vi "split string.vi"(10 "tokens":T4[](array[typedef]), 11 "String":string) -> (3 "layers":T1[](array[typedef]))   [LabVIEW 2013]
uses:
  json token.ctl
  json node type.ctl
  layer.ctl
  processed node.ctl
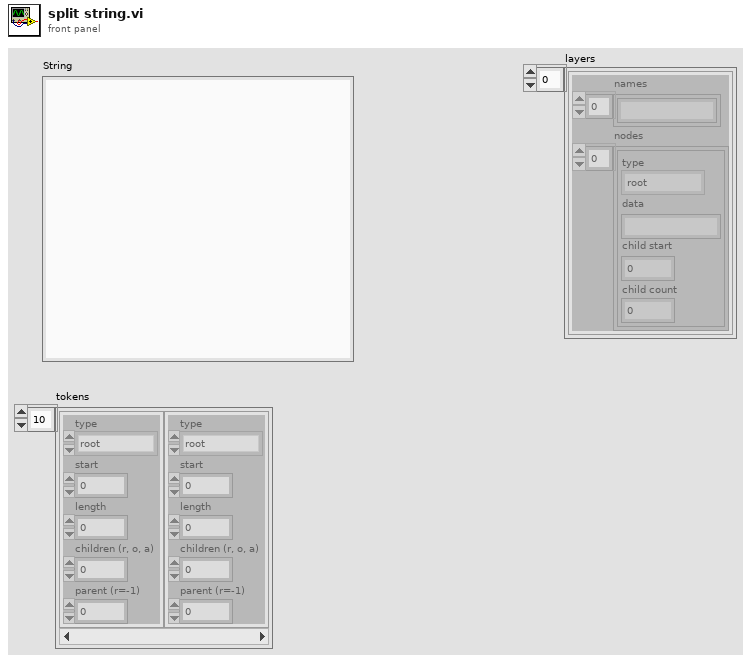
[diagram p1: front panel]
types:
  T1 = typedef "layer.ctl" = cluster{"names":string[], "nodes":T2[]}
  T2 = typedef "processed node.ctl" = cluster{"type":T3, "data":string, "child start":i32, "child count":i32}
  T3 = typedef "json node type.ctl" = enum16{"root", "object", "array", "number", "string value", "string key", "true", "false", "null"}
  T4 = typedef "json token.ctl" = cluster{"type":T3, "start":i32, "length":i32, "children (r, o, a)":u16, "parent (r=-1)":i32}
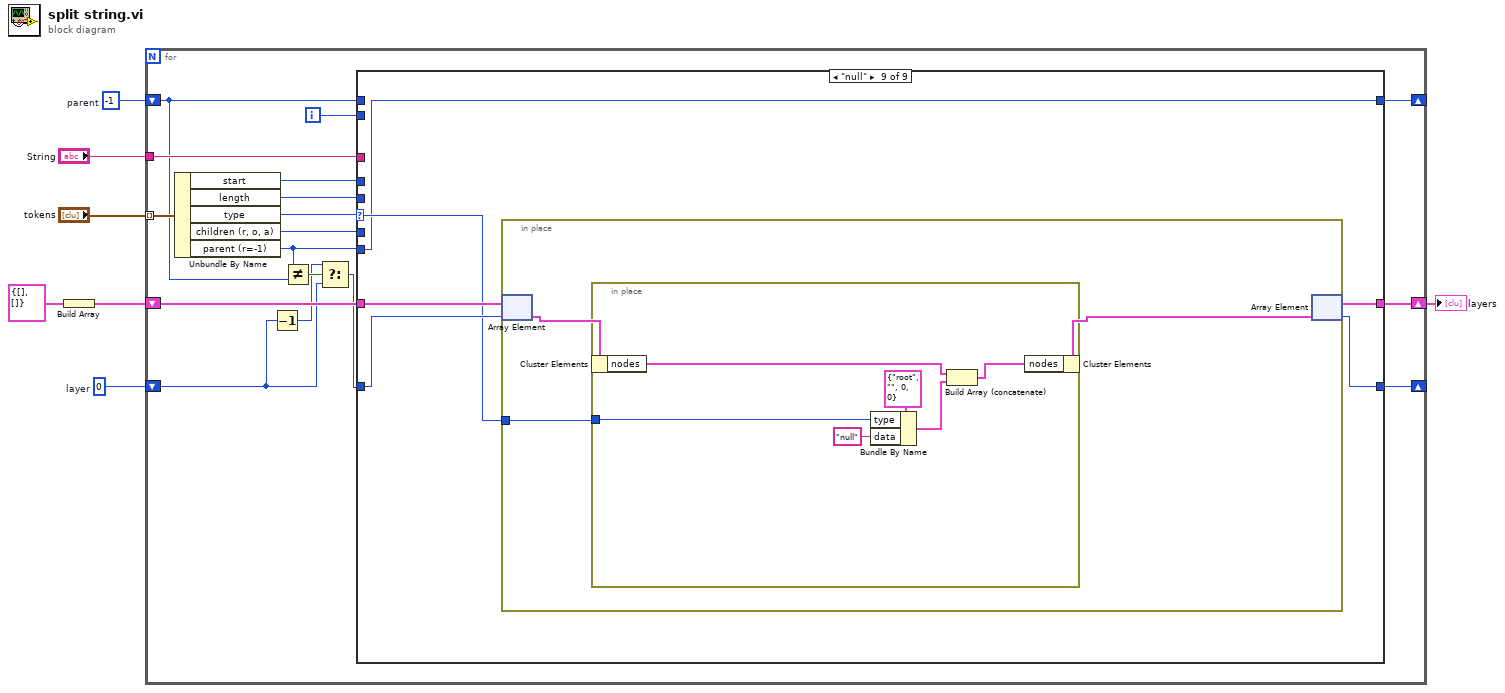
[diagram p0: block diagram]
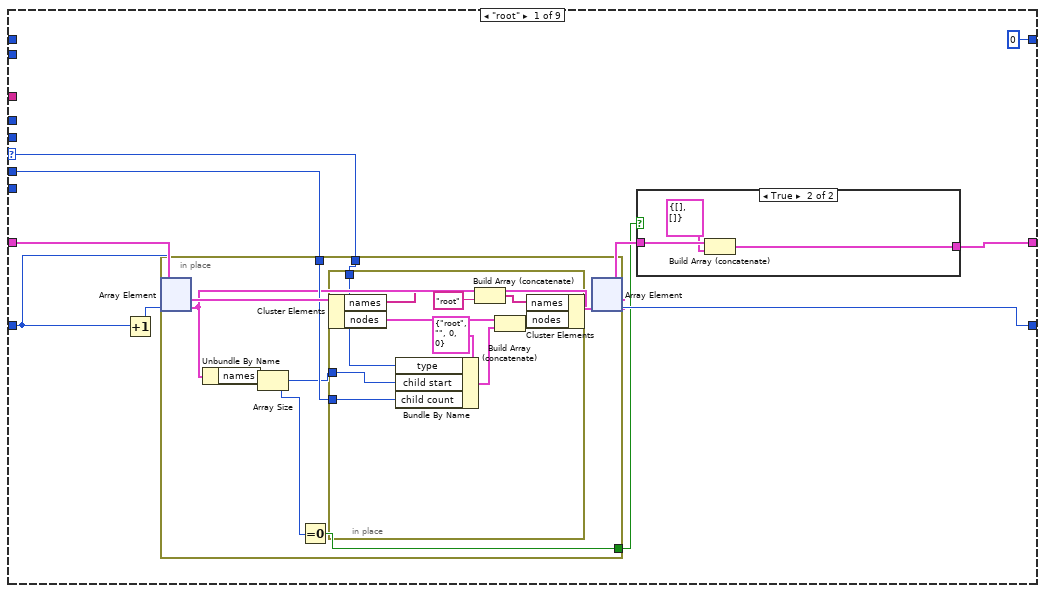
[diagram p2: hidden frame]
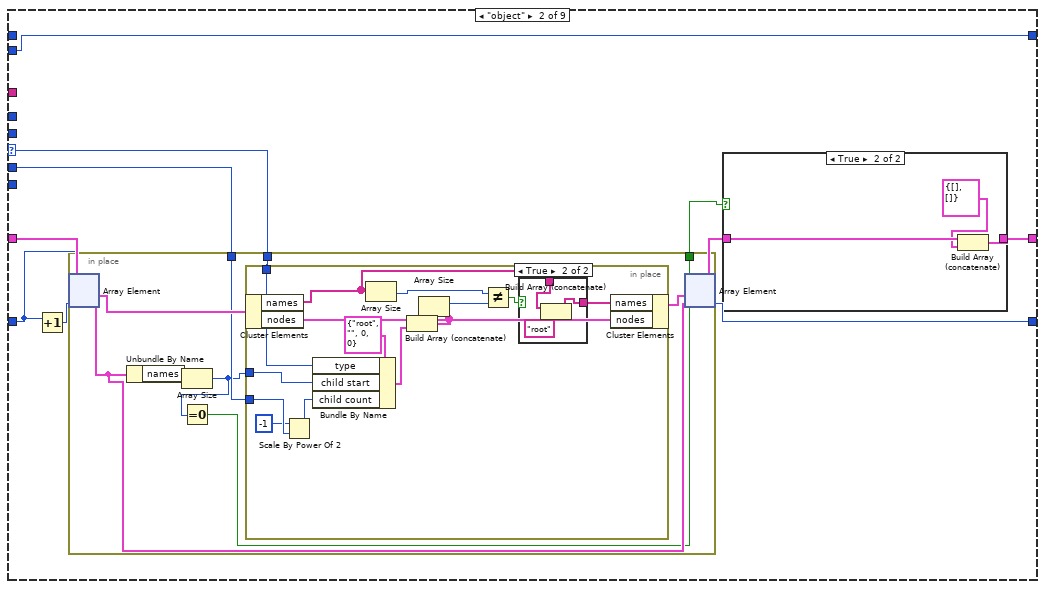
[diagram p4: hidden frame]
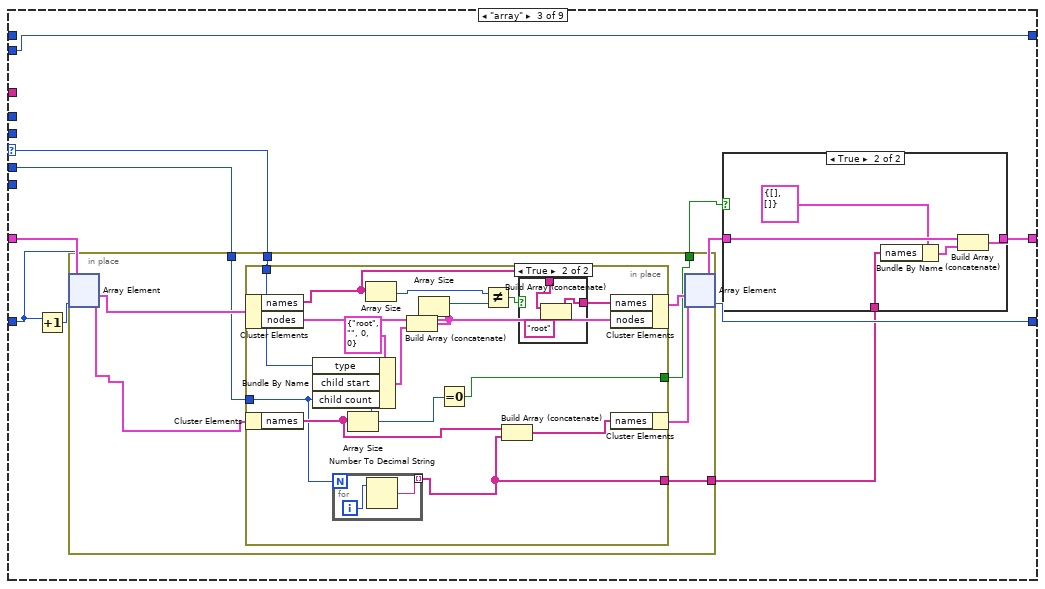
[diagram p7: hidden frame]
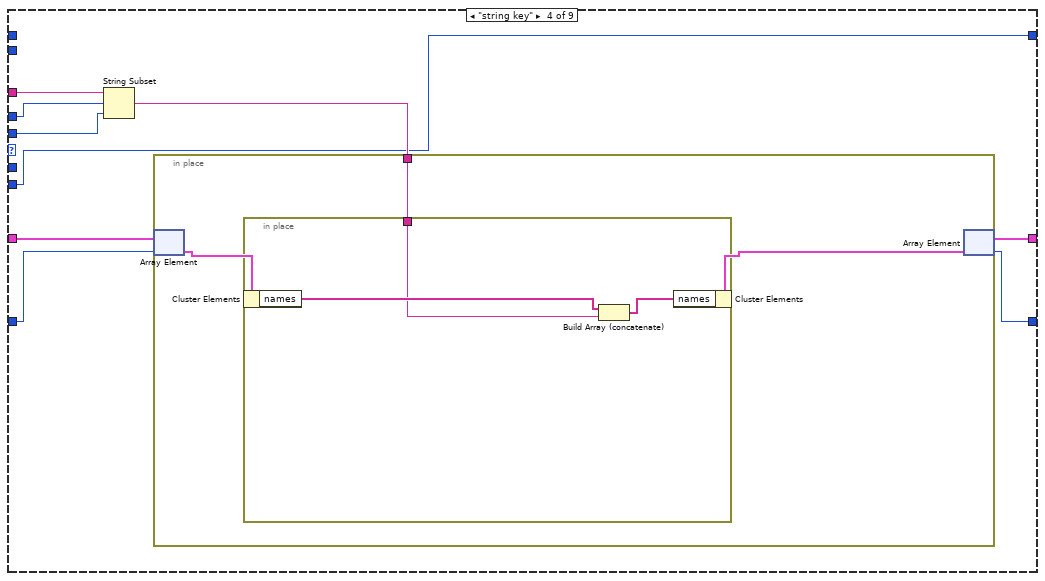
[diagram p10: hidden frame]
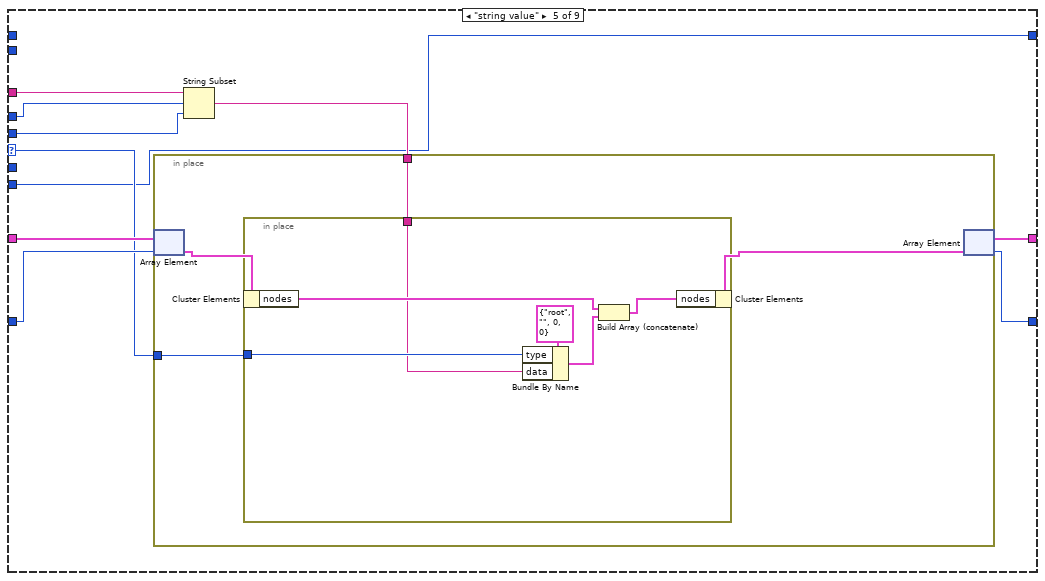
[diagram p11: hidden frame]
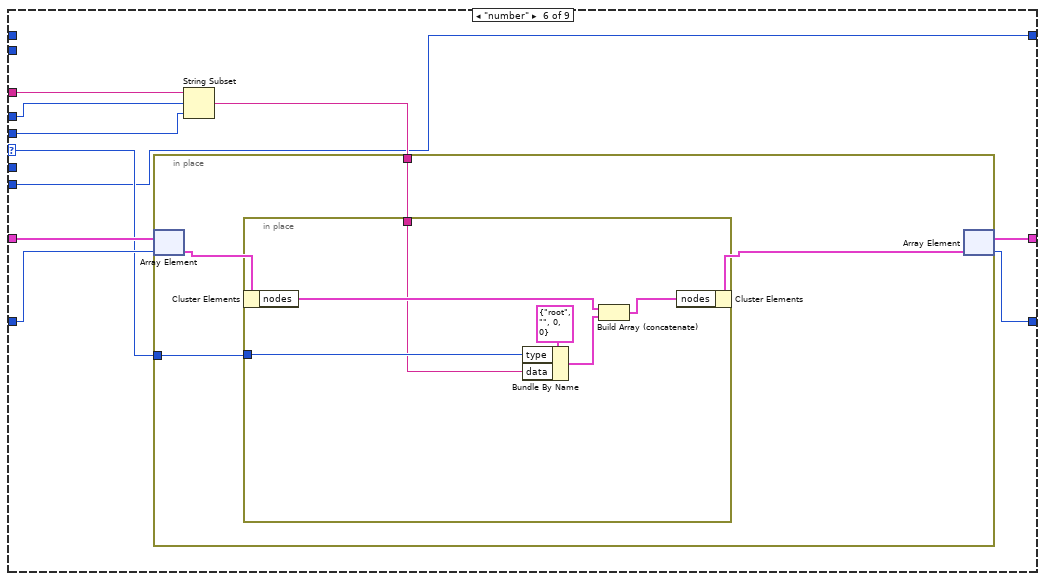
[diagram p12: hidden frame]
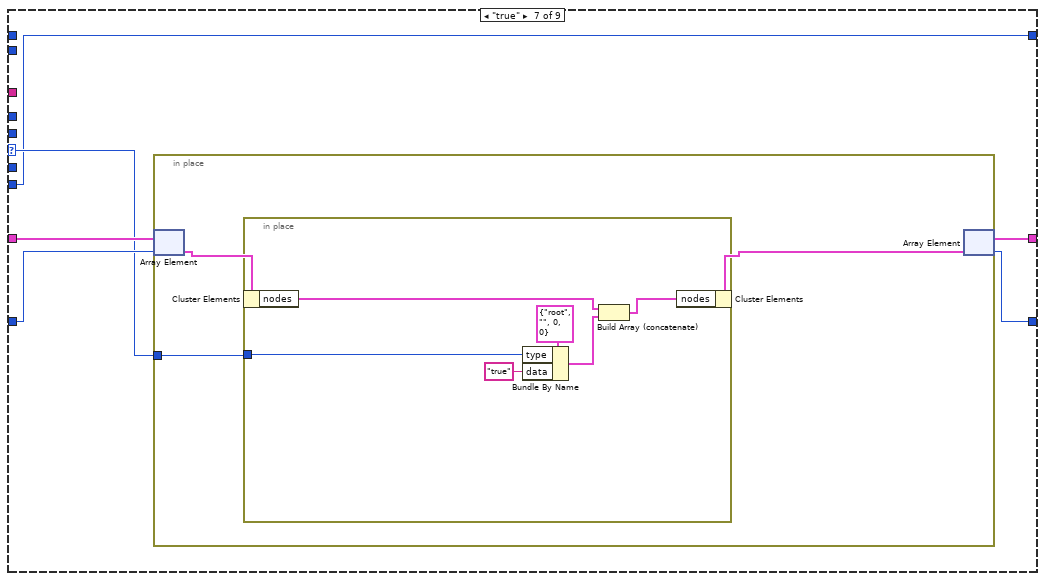
[diagram p13: hidden frame]
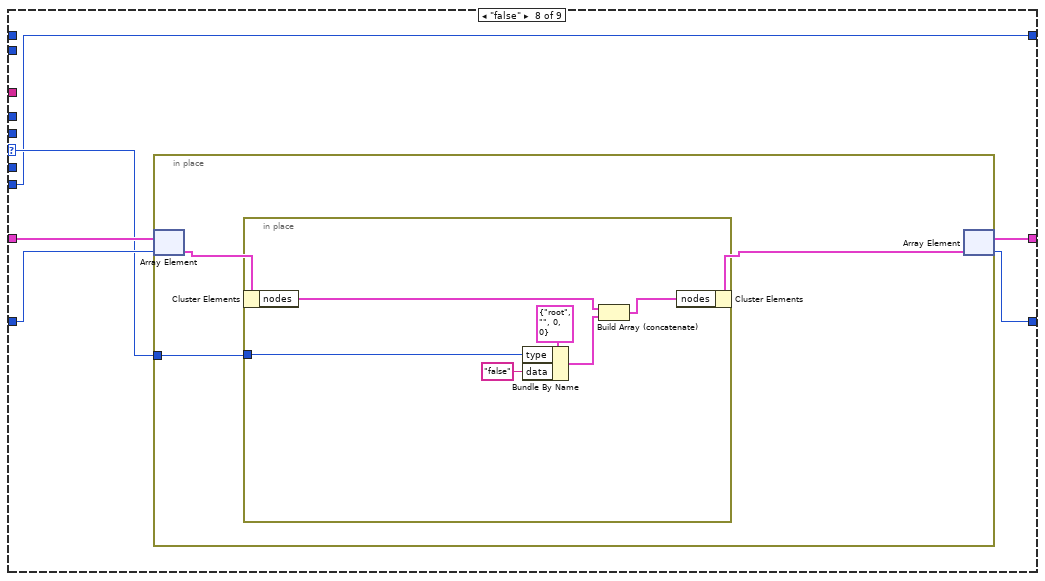
[diagram p14: hidden frame]
diagram:
  w3 = -1  # parent
  w4 = 0  # layer
  n1 = Build Array(T1 {"names"=[], "nodes"=[]} ("layer")) -> (w1:T1[])
  n2 = for {
    tunnel: "tokens" -> [w24] mode=indexing
    tunnel: "String" -> [w22]
    shift-right: [w17] -> w5
    shift-left: w1 -> [w18]
    shift-right: [w16] -> _
    shift-left: w4 -> [w10]
    shift-right: [w15] -> _
    shift-left: w3 -> [w13]
    i -> [w8]
    n3 = Unbundle By Name(w24) -> ("start"=w21:i32, "length"=w19:i32, "type"=w23:T3, "children (r, o, a)"=w20:u16, "parent (r=-1)"=w14:i32)
    n4 = Decrement(x=w10) -> (x-1=w11:i32)
    n5 = Not Equal?(x=w14, y=w13) -> (x != y?=w12:bool)
    n6 = Select(t=w11, s=w12, f=w10) -> (s? t:f=w9:i32)
    n7 = case shown="\"null\"" w23 {
      selector: w23 -> [w29 w61 w102 _ w164 w184 w200 w215 w230]
      tunnel: w22 -> [_ _ _ w148 w163 w183 _ _ _]
      tunnel: w21 -> [_ _ _ w147 w162 w182 _ _ _]
      tunnel: w20 -> [w28 w60 w101 _ _ _ _ _ _]
      tunnel: w19 -> [_ _ _ w146 w161 w181 _ _ _]
      tunnel: w14 -> [_ _ _ w144 w159 w179 w199 w214 w229]
      tunnel: w18 -> [w34 w66 w107 w151 w167 w187 w203 w218 w233]
      tunnel: w9 -> [w32 w64 w105 w152 w168 w188 w204 w219 w234]
      tunnel: [w26 w58 w99 w150 w166 w186 w202 w217 w232] -> w17
      tunnel: [w30 w62 w103 w149 w165 w185 w201 w216 w231] -> w16
      tunnel: [0 ("parent") w59 w100 w144 w159 w179 w199 w214 w229] -> w15
      tunnel: w13 -> [_ _ _ _ _ _ _ _ _]
      tunnel: w8 -> [_ w59 w100 _ _ _ _ _ _]
      frame "root" {
        n8 = Increment(x=w32) -> (x+1=w31:i32)
        n9 = in-place {
          in-place-border: w29 -> [w44]
          in-place-border: w28 -> [w43]
          in-place-border: [w39] -> w25
          n10 = in-place-array #1(w34, w32, w31) -> (w46:T1, w41:T1)
          n11 = Unbundle By Name(w41) -> ("names"=w42:string[])
          n12 = Array Size(array=w42) -> (size(s)=w40:i32)
          n13 = Equal To 0?(x=w40) -> (x = 0?=w39:bool)
          n14 = in-place {
            in-place-border: w44 -> [w50]
            in-place-border: w43 -> [w48]
            in-place-border: w40 -> [w47]
            n15 = in-place-cluster #2(w46) -> ("names"=w56:string[], "nodes"=w53:T2[])
            n16 = Bundle By Name(cluster=T2 {"type"=enum."root", "data"="", "child start"=0, "child count"=0} ("node"), "type"=w50, "child start"=w47, "child count"=w48) -> (w49:T2)
            n17 = Build Array (concatenate)(w56, "root") -> (w54:string[])
            n18 = Build Array (concatenate)(w53, w49) -> (w52:T2[])
            n19 = in-place-cluster #2("names"=w54, "nodes"=w52) -> (w45:T1)
          }
          n20 = in-place-array #1(w45, w41) -> (w33:T1[], w30:i32)  [unwired: 1 out]
        }
        n21 = case shown="True" w25 {
          tunnel: w33 -> [w35 w38]
          tunnel: [w35 w37] -> w26
          frame False {
          }
          frame True {
            n22 = Build Array (concatenate)(w38, T1 {"names"=[], "nodes"=[]} ("layer")) -> (w37:T1[])
          }
        }
      }
      frame "object" {
        n23 = Increment(x=w64) -> (x+1=w63:i32)
        n24 = in-place {
          in-place-border: w61 -> [w76]
          in-place-border: w60 -> [w75]
          in-place-border: [w71] -> w57
          n25 = in-place-array #3(w66, w64, w63) -> (w78:T1, w73:T1)
          n26 = Unbundle By Name(w73) -> ("names"=w74:string[])
          n27 = Array Size(array=w74) -> (size(s)=w72:i32)
          n28 = Equal To 0?(x=w72) -> (x = 0?=w71:bool)
          n29 = in-place {
            in-place-border: w76 -> [w90]
            in-place-border: w75 -> [w81]
            in-place-border: w72 -> [w88]
            n30 = in-place-cluster #4(w78) -> ("names"=w83:string[], "nodes"=w92:T2[])
            n31 = Scale By Power Of 2(n=i16 -1, x=w81) -> (x*2^n=w80:u16)
            n32 = Bundle By Name(cluster=T2 {"type"=enum."root", "data"="", "child start"=0, "child count"=0} ("node"), "type"=w90, "child start"=w88, "child count"=w80) -> (w89:T2)
            n33 = Array Size(array=w83) -> (size(s)=w85:i32)
            n34 = Build Array (concatenate)(w92, w89) -> (w87:T2[])
            n35 = Array Size(array=w87) -> (size(s)=w86:i32)
            n36 = Not Equal?(x=w85, y=w86) -> (x != y?=w84:bool)
            n37 = case shown="True" w84 {
              tunnel: w83 -> [w93 w96]
              tunnel: [w93 w95] -> w82
              frame False {
              }
              frame True {
                n38 = Build Array (concatenate)(w96, "root") -> (w95:string[])
              }
            }
            n39 = in-place-cluster #4("names"=w82, "nodes"=w87) -> (w77:T1)
          }
          n40 = in-place-array #3(w77, w73) -> (w65:T1[], w62:i32)  [unwired: 1 out]
        }
        n41 = case shown="True" w57 {
          tunnel: w65 -> [w67 w70]
          tunnel: [w67 w69] -> w58
          frame False {
          }
          frame True {
            n42 = Build Array (concatenate)(w70, T1 {"names"=[], "nodes"=[]} ("layer")) -> (w69:T1[])
          }
        }
      }
      frame "array" {
        n43 = Increment(x=w105) -> (x+1=w104:i32)
        n44 = in-place {
          in-place-border: w102 -> [w119]
          in-place-border: w101 -> [w118]
          in-place-border: [w115] -> w98
          in-place-border: [w114] -> w97
          n45 = in-place-array #5(w107, w105, w104) -> (w121:T1, w117:T1)
          n46 = in-place {
            in-place-border: w119 -> [w135]
            in-place-border: w118 -> [w123]
            in-place-border: [w127] -> w115
            in-place-border: [w122] -> w114
            n47 = in-place-cluster #6(w121) -> ("names"=w129:string[], "nodes"=w137:T2[])
            n48 = in-place-cluster #7(w117) -> ("names"=w125:string[])
            n49 = for {
              N: w123 -> [_]
              tunnel: [w138] -> w122 mode=indexing
              i -> [w139]
              n50 = Number To Decimal String(number=w139) -> (decimal integer string=w138:string)  [unwired: 1 in]
            }
            n51 = Array Size(array=w125) -> (size(s)=w126:i32)
            n52 = Bundle By Name(cluster=T2 {"type"=enum."root", "data"="", "child start"=0, "child count"=0} ("node"), "type"=w135, "child start"=w126, "child count"=w123) -> (w134:T2)
            n53 = Array Size(array=w129) -> (size(s)=w131:i32)
            n54 = Build Array (concatenate)(w137, w134) -> (w133:T2[])
            n55 = Array Size(array=w133) -> (size(s)=w132:i32)
            n56 = Equal To 0?(x=w126) -> (x = 0?=w127:bool)
            n57 = Not Equal?(x=w131, y=w132) -> (x != y?=w130:bool)
            n58 = Build Array (concatenate)(w125, w122) -> (w124:string[])
            n59 = case shown="True" w130 {
              tunnel: w129 -> [w140 w143]
              tunnel: [w140 w142] -> w128
              frame False {
              }
              frame True {
                n60 = Build Array (concatenate)(w143, "root") -> (w142:string[])
              }
            }
            n61 = in-place-cluster #6("names"=w128, "nodes"=w133) -> (w120:T1)
            n62 = in-place-cluster #7("names"=w124) -> (w116:T1)
          }
          n63 = in-place-array #5(w120, w116) -> (w106:T1[], w103:i32)  [unwired: 1 out]
        }
        n64 = case shown="True" w98 {
          tunnel: w106 -> [w108 w113]
          tunnel: [w108 w112] -> w99
          tunnel: w97 -> [_ w109]
          frame False {
          }
          frame True {
            n65 = Bundle By Name(cluster=T1 {"names"=[], "nodes"=[]} ("layer"), "names"=w109) -> (w110:T1)
            n66 = Build Array (concatenate)(w113, w110) -> (w112:T1[])
          }
        }
      }
      frame "string key" {
        n67 = String Subset(string=w148, offset (0)=w147, length (rest)=w146) -> (substring=w145:string)
        n68 = in-place {
          in-place-border: w145 -> [w153]
          n69 = in-place-array #8(w151, w152) -> (w155:T1)
          n70 = in-place {
            in-place-border: w153 -> [w156]
            n71 = in-place-cluster #9(w155) -> ("names"=w158:string[])
            n72 = Build Array (concatenate)(w158, w156) -> (w157:string[])
            n73 = in-place-cluster #9("names"=w157) -> (w154:T1)
          }
          n74 = in-place-array #8(w154) -> (w150:T1[], w149:i32)
        }
      }
      frame "string value" {
        n75 = String Subset(string=w163, offset (0)=w162, length (rest)=w161) -> (substring=w160:string)
        n76 = in-place {
          in-place-border: w164 -> [w170]
          in-place-border: w160 -> [w169]
          n77 = in-place-array #10(w167, w168) -> (w172:T1)
          n78 = in-place {
            in-place-border: w170 -> [w174]
            in-place-border: w169 -> [w173]
            n79 = in-place-cluster #11(w172) -> ("nodes"=w176:T2[])
            n80 = Bundle By Name(cluster=T2 {"type"=enum."root", "data"="", "child start"=0, "child count"=0} ("node"), "type"=w174, "data"=w173) -> (w178:T2)
            n81 = Build Array (concatenate)(w176, w178) -> (w175:T2[])
            n82 = in-place-cluster #11("nodes"=w175) -> (w171:T1)
          }
          n83 = in-place-array #10(w171) -> (w166:T1[], w165:i32)
        }
      }
      frame "number" {
        n84 = String Subset(string=w183, offset (0)=w182, length (rest)=w181) -> (substring=w180:string)
        n85 = in-place {
          in-place-border: w184 -> [w190]
          in-place-border: w180 -> [w189]
          n86 = in-place-array #12(w187, w188) -> (w192:T1)
          n87 = in-place {
            in-place-border: w190 -> [w194]
            in-place-border: w189 -> [w193]
            n88 = in-place-cluster #13(w192) -> ("nodes"=w196:T2[])
            n89 = Bundle By Name(cluster=T2 {"type"=enum."root", "data"="", "child start"=0, "child count"=0} ("node"), "type"=w194, "data"=w193) -> (w198:T2)
            n90 = Build Array (concatenate)(w196, w198) -> (w195:T2[])
            n91 = in-place-cluster #13("nodes"=w195) -> (w191:T1)
          }
          n92 = in-place-array #12(w191) -> (w186:T1[], w185:i32)
        }
      }
      frame "true" {
        n93 = in-place {
          in-place-border: w200 -> [w205]
          n94 = in-place-array #14(w203, w204) -> (w207:T1)
          n95 = in-place {
            in-place-border: w205 -> [w209]
            n96 = in-place-cluster #15(w207) -> ("nodes"=w211:T2[])
            n97 = Bundle By Name(cluster=T2 {"type"=enum."root", "data"="", "child start"=0, "child count"=0} ("node"), "type"=w209, "data"="true") -> (w213:T2)
            n98 = Build Array (concatenate)(w211, w213) -> (w210:T2[])
            n99 = in-place-cluster #15("nodes"=w210) -> (w206:T1)
          }
          n100 = in-place-array #14(w206) -> (w202:T1[], w201:i32)
        }
      }
      frame "false" {
        n101 = in-place {
          in-place-border: w215 -> [w220]
          n102 = in-place-array #16(w218, w219) -> (w222:T1)
          n103 = in-place {
            in-place-border: w220 -> [w224]
            n104 = in-place-cluster #17(w222) -> ("nodes"=w226:T2[])
            n105 = Bundle By Name(cluster=T2 {"type"=enum."root", "data"="", "child start"=0, "child count"=0} ("node"), "type"=w224, "data"="false") -> (w228:T2)
            n106 = Build Array (concatenate)(w226, w228) -> (w225:T2[])
            n107 = in-place-cluster #17("nodes"=w225) -> (w221:T1)
          }
          n108 = in-place-array #16(w221) -> (w217:T1[], w216:i32)
        }
      }
      frame "null" {
        n109 = in-place {
          in-place-border: w230 -> [w235]
          n110 = in-place-array #18(w233, w234) -> (w237:T1)
          n111 = in-place {
            in-place-border: w235 -> [w239]
            n112 = in-place-cluster #19(w237) -> ("nodes"=w241:T2[])
            n113 = Bundle By Name(cluster=T2 {"type"=enum."root", "data"="", "child start"=0, "child count"=0} ("node"), "type"=w239, "data"="null") -> (w243:T2)
            n114 = Build Array (concatenate)(w241, w243) -> (w240:T2[])
            n115 = in-place-cluster #19("nodes"=w240) -> (w236:T1)
          }
          n116 = in-place-array #18(w236) -> (w232:T1[], w231:i32)
        }
      }
    }
  }
  "layers" <- w5
